vi "Read Data.vi"(8 "error in (no error)":errorcluster, 11 "Test Station SIM AI Driver in":refnum<class "Test Station SIM AI Driver.lvclass">) -> (0 "error out":errorcluster, 2 "Daq Data":T1, 3 "Test Station SIM AI Driver out":refnum<class "Test Station SIM AI Driver.lvclass">)   [LabVIEW 2022 SP3, in "Test Station SIM AI Driver.lvclass"]
uses:
  Test Station SIM AI Driver.lvclass
  DAQ Data/AIDAQ Data.ctl
  Laser/Test Station SIM Laser Driver/Action.ctl
  Test Station SIM AI Driver.lvclass/Test Station SIM AI Driver.ctl
  DAQ Data/AI Daq Data.lvlib
  Laser/Test Station SIM Laser Driver/Test Station SIM Laser Driver.lvclass
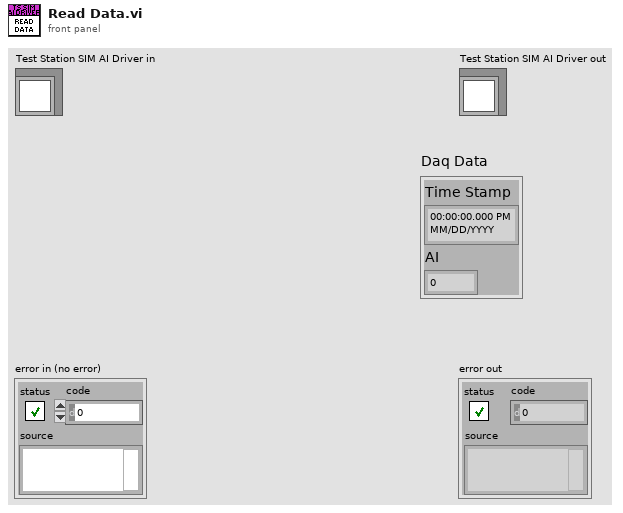
[diagram p1: front panel]
types:
  T1 = typedef "AI Daq Data.lvlib/AIDAQ Data.ctl" = cluster{"Time Stamp":timestamp, "AI":dbl}
  T2 = typedef "Test Station SIM Laser Driver.lvclass/Action.ctl" = enum16{"Read Data", "Set Data"}
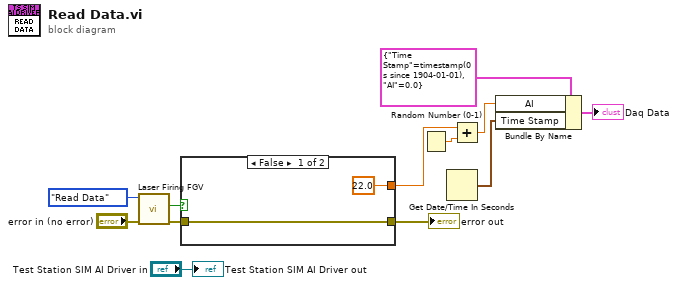
[diagram p0: block diagram]
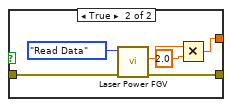
[diagram p2: hidden frame]
diagram:
  n1 = call "Laser Firing FGV.vi"("error in (no error)"="error in (no error)", "Action"=Action."Read Data") -> ("error out"=w3:errorcluster, "Laser Firing"=w5:bool)  [unwired: 8 in]
  n2 = case shown="False" w5 {
    tunnel: [22.0 w18] -> w6
    tunnel: w3 -> [w13 w16]
    tunnel: [w13 w15] -> w1
    frame False {
    }
    frame True {
      n3 = call "Laser Power FGV.vi"("error in (no error)"=w16, "Action"=Action."Read Data") -> ("error out"=w15:errorcluster, "Laser Power"=w19:dbl)  [unwired: 8 in]
      n4 = Multiply(x=w19, y=2.0) -> (x*y=w18:dbl)
    }
  }
  "error out" <- w1
  n5 = Random Number (0-1)() -> (number: 0 to 1=w7:dbl)
  n6 = Get Date/Time In Seconds() -> (seconds since 1Jan1904=w10:timestamp)
  n7 = Add(x=w6, y=w7) -> (x+y=w9:dbl)
  n8 = Bundle By Name(cluster=T1 {"Time Stamp"=timestamp(0 s since 1904-01-01), "AI"=0.0} ("Daq Data"), "AI"=w9, "Time Stamp"=w10) -> (→"Daq Data":T1)
  "Test Station SIM AI Driver out" <- "Test Station SIM AI Driver in"
